vi "GetPatterns.vi"(8 "Error In":errorcluster {"code" format="%.0x"}, 11 "Cards In":cluster{"Session":u32, "Card number":u32}[](array[cluster])) -> (0 "Error Out":errorcluster, 2 "Patterns":T1[](array[typedef]), 3 "Cards Out":cluster{"Session":u32, "Card number":u32}[](array[cluster]))   [LabVIEW 2012, in "Virtual-PGA.lvlib"]
uses:
  Virtual-PGA.lvlib
  Controls/Pattern.ctl
  Controls/Input.ctl
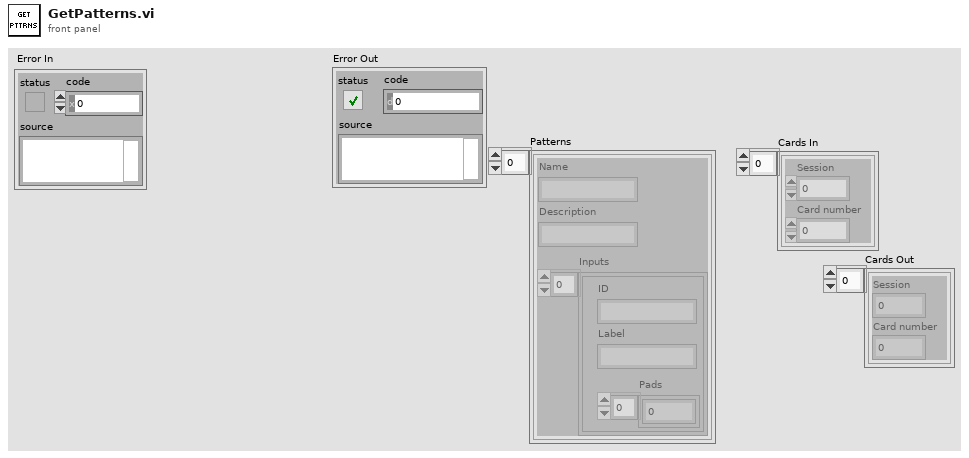
[diagram p1: front panel]
types:
  T1 = typedef "Virtual-PGA.lvlib/Pattern.ctl" = cluster{"Name":string, "Description":string, "Inputs":T2[]}
  T2 = typedef "Virtual-PGA.lvlib/Input.ctl" = cluster{"ID":string, "Label":string, "Pads":u32[]}
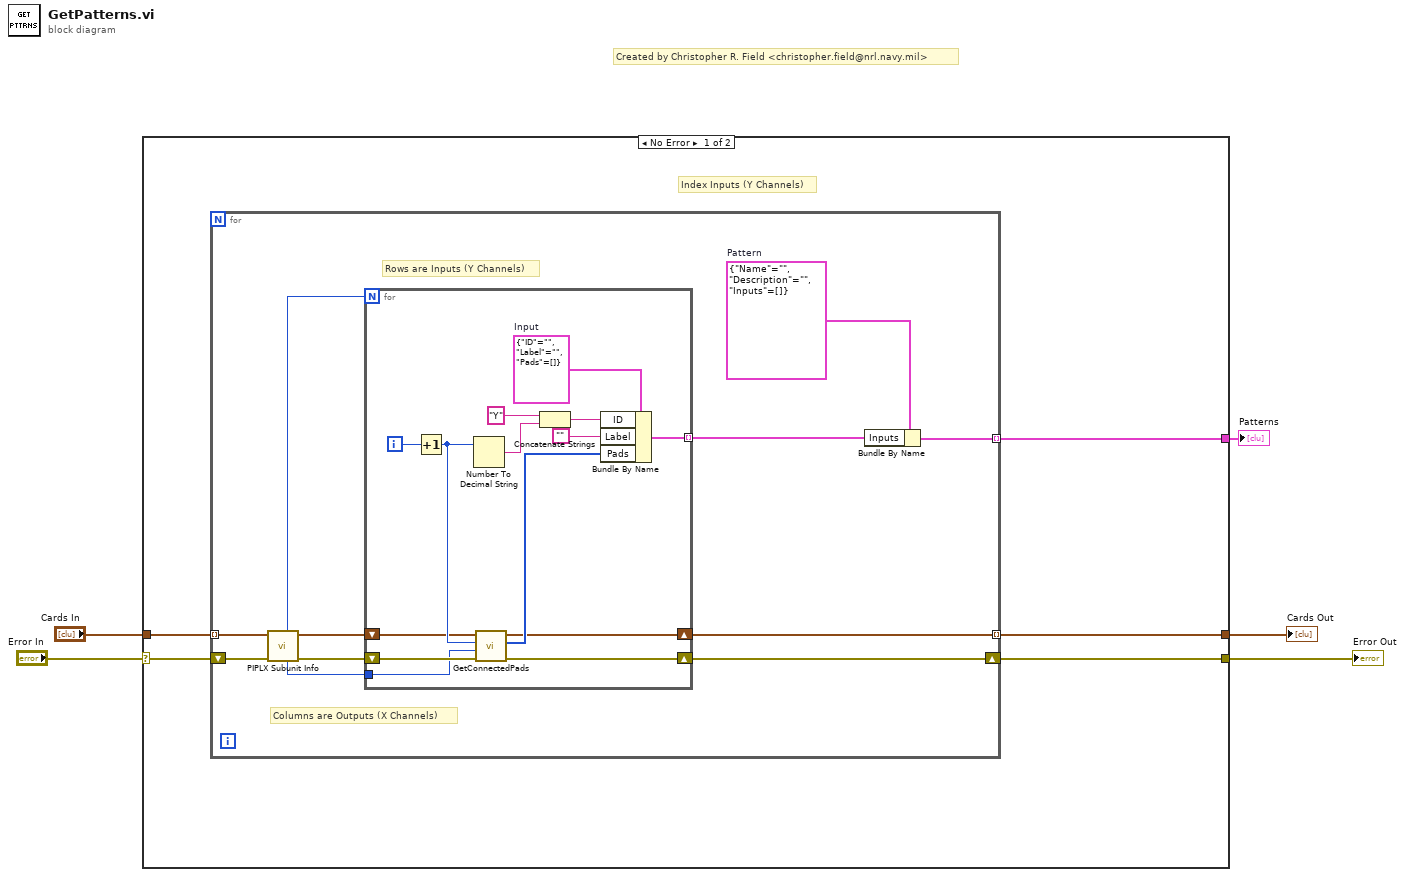
[diagram p0: block diagram]
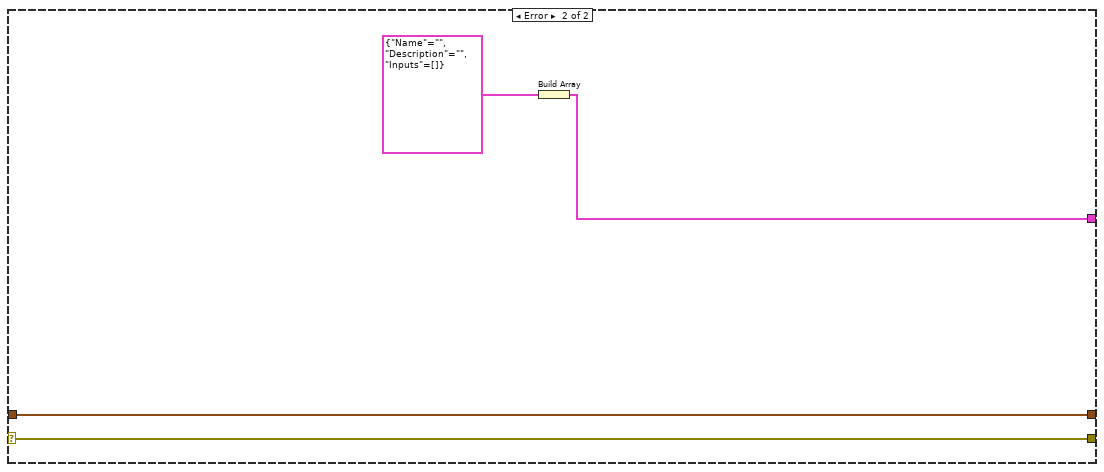
[diagram p2: hidden frame]
diagram:
  # "Created by Christopher R. Field <christopher.field@nrl.navy.mil>"
  n1 = case shown="No Error" "Error In" {
    selector: "Error In" -> [w10 w39]
    tunnel: [w8 w39] -> w5
    tunnel: "Cards In" -> [w9 w36]
    tunnel: [w6 w37] -> w2
    tunnel: [w7 w36] -> w1
    frame No Error {
      # "Index Inputs (Y Channels)"
      n2 = for {
        shift-right: [w14] -> w8
        shift-left: w10 -> [w20]
        tunnel: w9 -> [w21] mode=indexing
        tunnel: [w15] -> w7 mode=indexing
        tunnel: [w11] -> w6 mode=indexing
        w13 = T1 {"Name"="", "Description"="", "Inputs"=[]}  # Pattern
        # "Rows are Inputs (Y Channels)"
        # "Columns are Outputs (X Channels)"
        n3 = call <instrlib>:"PIPLX Subunit Info.vi"("error in"=w20, "Input Handle"=w21) -> ("error out"=w19:errorcluster, "Output Handle"=w18:cluster{"Session":u32, "Card number":u32}, "Columns"=w16:u32, "Rows"=w17:u32)  [unwired: 5 in, 1 out]
        n4 = for {
          N: w17 -> [_]
          tunnel: [w29] -> w12 mode=indexing
          shift-right: [w26] -> w14
          shift-left: w19 -> [w28]
          tunnel: w16 -> [w24]
          shift-right: [w22] -> w15
          shift-left: w18 -> [w25]
          i -> [w35]
          w32 = T2 {"ID"="", "Label"="", "Pads"=[]}  # Input
          n5 = Increment(x=w35) -> (x+1=w27:i32)
          n6 = Number To Decimal String(number=w27) -> (decimal integer string=w33:string)  [unwired: 1 in]
          n7 = call "GetConnectedPads.vi"("Error In"=w28, "Pad Number"=w24, "Input Index"=w27, "Card In"=w25) -> ("Error Out"=w26:errorcluster, "Pads"=w23:u32[], "Card Out"=w22:cluster{"Session":u32, "Card number":u32})  [unwired: 5 in]
          n8 = Concatenate Strings("Y", w33) -> (w31:string)
          n9 = Bundle By Name(cluster=w32, "ID"=w31, "Label"="", "Pads"=w23) -> (w29:T2)
        }
        n10 = Bundle By Name(cluster=w13, "Inputs"=w12) -> (w11:T1)
      }
    }
    frame Error {
      n11 = Build Array(T1 {"Name"="", "Description"="", "Inputs"=[]} ("Pattern")) -> (w37:T1[])
    }
  }
  "Error Out" <- w5
  "Cards Out" <- w1
  "Patterns" <- w2
